vi "test_unpacking.vi"() -> ()   [LabVIEW 2023]
uses:
  HoloPyLib/holoPyTracks.lvlib
  HologramInfo.ctl
  analyse_parameters.ctl
  HoloPyLib/CCL_parameters.ctl
panel:
  out "return value 2":string
  in  "analyse parameters":T1={"propagation"={"distance ini"=0.0, "number of planes"=0, "step"=0.0, "Fourier BP filter (pix)"={"High pass (0=none)"=0.0, "Low Pass (0=none)"=0.0}}, "Focus"={"Type"=enum."SUM_OF_INTENSITY", "Sum size"=1}, "Remove mean Hologram"=FALSE, "CCL parameters"={"Threshold ( N x Standard deviation)"=10.0, "Connectivity"=enum."6", "min voxel"=1.0, "max voxel"=1.0}} {"CCL parameters"."max voxel" min=0.0 max=0.0; "CCL parameters"."min voxel" min=1.0 max=100.0; "CCL parameters"."Threshold ( N x Standard deviation)" min=1.0 max=100.0; "Focus"."Sum size" min=1 max=100; "propagation"."Fourier BP filter (pix)"."Low Pass (0=none)" format="%#_6e"; "propagation"."step" format="%#_6e"; "propagation"."distance ini" format="%#_6e"}
  in  "Holo parameters":T3 {"Holo size X" format="%#_6e"; "wavelength" format="%#_6e"}
  out "return value":sgl[][](array[numeric])
  in  "image path":path
  in  "error in (no error)":errorcluster
  in  "Python version":string="3.10"
  out "error out":errorcluster
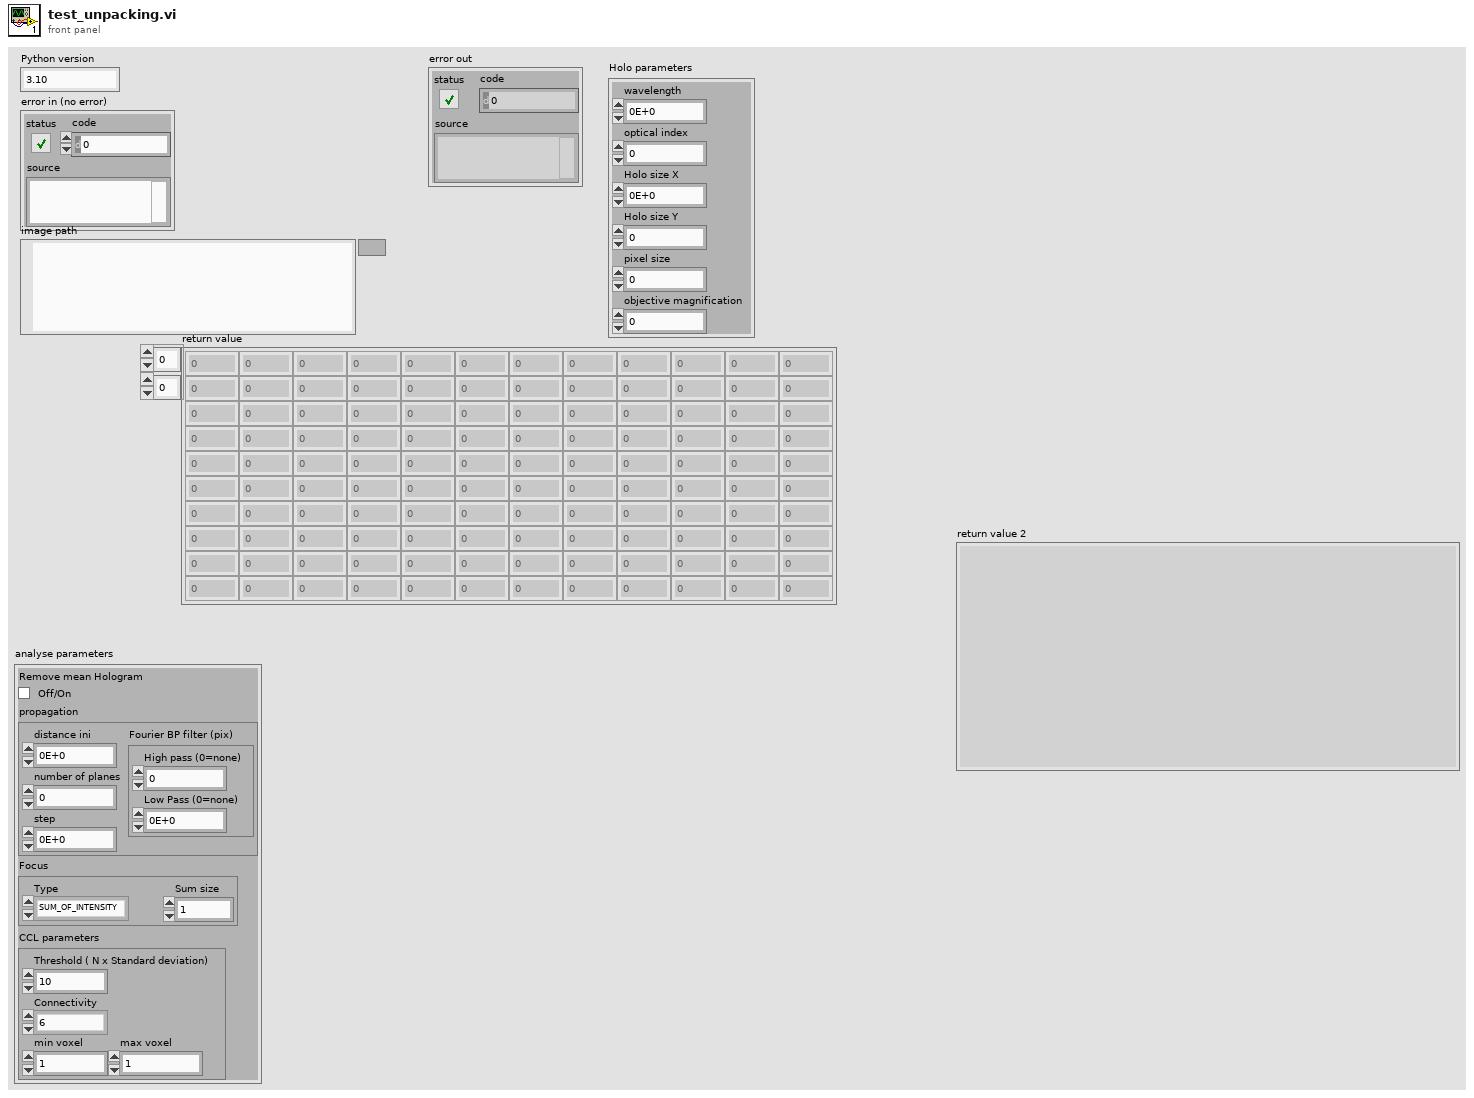
[diagram p1: front panel]
types:
  T1 = typedef "holoPyTracks.lvlib/analyse_parameters.ctl" = cluster{"propagation":cluster{"distance ini":dbl, "number of planes":i32, "step":dbl, "Fourier BP filter (pix)":cluster{"High pass (0=none)":dbl, "Low Pass (0=none)":dbl}}, "Focus":cluster{"Type":enum16{"SUM_OF_INTENSITY", "SUM_OF_LAPLACIAN", "SUM_OF_VARIANCE", "TENENGRAD"}, "Sum size":i32}, "Remove mean Hologram":bool, "CCL parameters":T2}
  T2 = typedef "CCL_parameters.ctl" = cluster{"Threshold ( N x Standard deviation)":dbl, "Connectivity":enum16{"6", "18", "26"}, "min voxel":dbl, "max voxel":dbl}
  T3 = typedef "holoPyTracks.lvlib/HologramInfo.ctl" = cluster{"wavelength":sgl, "optical index":sgl, "Holo size X":i32, "Holo size Y":i32, "pixel size":sgl, "objective magnification":sgl}
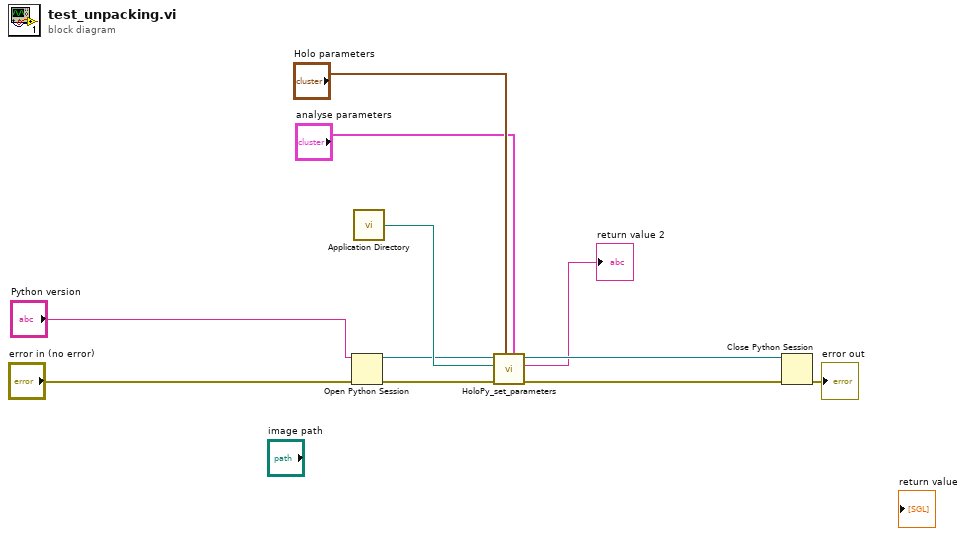
[diagram p0: block diagram]
diagram:
  n1 = Open Python Session(python version="Python version", 3:"error in (no error)") -> (session out=w2:refnum<k35>, error out=w1:errorcluster)  [unwired: 1 in]
  n2 = call <vilib>:"Application Directory.vi"() -> ("Application Directory"=w4:path)
  n3 = call "HoloPy_set_parameters.vi"(5:"analyse parameters", 7:"Holo parameters", "error in (no error)"=w1, "ParametersIN"=w4, "session in"=w2) -> ("error out"=w6:errorcluster, "return value"=→"return value 2":string, "Refnum out"=w5:refnum<k35>)  [unwired: 4 in]
  n4 = Close Python Session(session in=w5, error in=w6) -> (11:→"error out":errorcluster)
